vi "createNewPage.vi"(6 "Set as active (T)":bool=TRUE, 8 "error in (no error)":errorcluster, 10 "Page Name":string, 11 "MS-Excel in":refnum<class "MS-Excel.lvclass">) -> (0 "error out":errorcluster, 1 "Created?":bool, 2 "Created Page Name":string, 3 "MS-Excel out":refnum<class "MS-Excel.lvclass">)   [LabVIEW 2017, in "LabVIEW NPOI.lvlib" / "MS-Excel.lvclass"]
uses:
  MS-Excel.lvclass
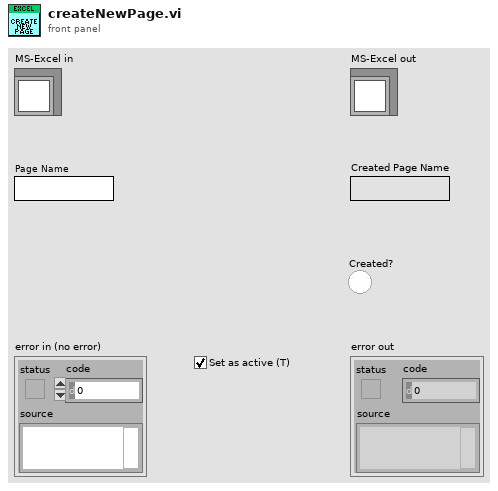
[diagram p1: front panel]
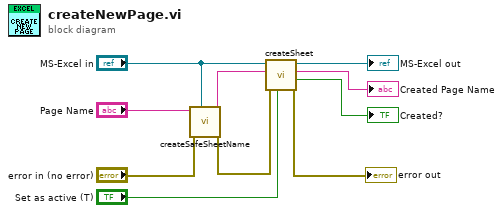
[diagram p0: block diagram]
diagram:
  n1 = call "createSafeSheetName.vi"("MS-Excel in"="MS-Excel in", "error in (no error)"="error in (no error)", "nameProposal"="Page Name") -> ("error out"=w9:errorcluster, "SafeSheetName"=w10:string)  [unwired: 7 in]
  n2 = call-dynamic "createSheet.vi"("Set as active (T)"="Set as active (T)", "error in (no error)"=w9, "SheetName"=w10, "MS-Excel in"="MS-Excel in") -> ("error out"=→"error out":errorcluster, "Created?"=→"Created?":bool, "Created Sheet Name"=→"Created Page Name":string, "MS-Excel out"=→"MS-Excel out":refnum<class "MS-Excel.lvclass">)  [unwired: 4 in]
